vi "SetGetUnits - Test.vi"() -> ()   [LabVIEW 2017]
uses:
  AT901 API/Structures/Struct SystemUnits.ctl
  AT901 API/TypeDefinitions/ES_LengthUnit.ctl
  AT901 API/TypeDefinitions/ES_AngleUnit.ctl
  AT901 API/TypeDefinitions/ES_TemperatureUnit.ctl
  AT901 API/TypeDefinitions/ES_PressureUnit.ctl
  AT901 API/TypeDefinitions/ES_HumidityUnit.ctl
panel:
  in  "SystemUnits 2":T1
  out "SystemUnits":T1
  out "error out":errorcluster
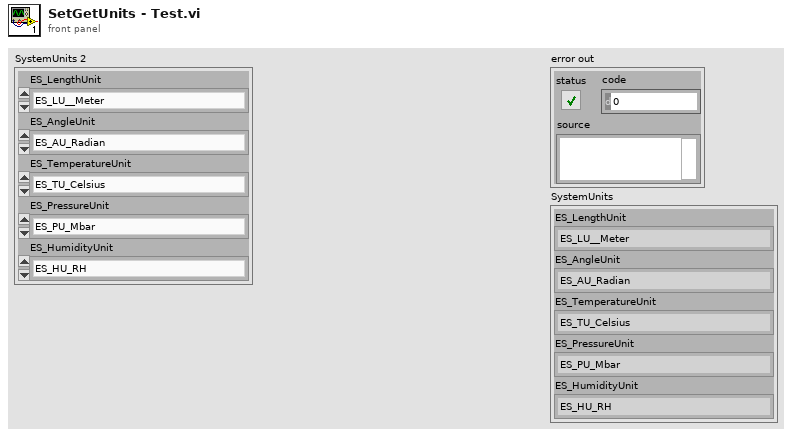
[diagram p1: front panel]
types:
  T1 = typedef "Struct SystemUnits.ctl" = cluster{"ES_LengthUnit":T2, "ES_AngleUnit":T3, "ES_TemperatureUnit":T4, "ES_PressureUnit":T5, "ES_HumidityUnit":T6}
  T2 = typedef "ES_LengthUnit.ctl" = enum32{"ES_LU__Meter", "ES_LU_Millimeter", "ES_LU_Micron", "ES_LU_Foot", "ES_LU_Yard", "ES_LU_Inch"}
  T3 = typedef "ES_AngleUnit.ctl" = enum32{"ES_AU_Radian", "ES_AU_Degree", "ES_AU_Gon"}
  T4 = typedef "ES_TemperatureUnit.ctl" = enum32{"ES_TU_Celsius", "ES_TU_Fahrenheit"}
  T5 = typedef "ES_PressureUnit.ctl" = enum32{"ES_PU_Mbar", "ES_PU_HPascal", "ES_PU_KPascal", "ES_PU_MmHg", "ES_PU_Psi", "ES_PU_InH2O", "ES_PU_InHg"}
  T6 = typedef "ES_HumidityUnit.ctl" = enum32{"ES_HU_RH"}
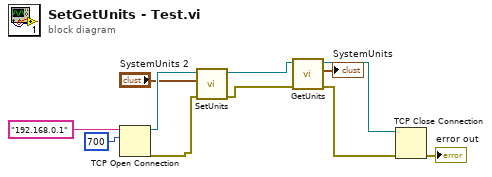
[diagram p0: block diagram]
diagram:
  n1 = TCP Open Connection(address="192.168.0.1", remote port or service name=u16 700) -> (connection ID=w3:refnum<k5>, error out=w8:errorcluster)  [unwired: 3 in]
  n2 = call "SetUnits.vi"("error in (no error)"=w8, "SystemUnits"="SystemUnits 2", "TCP Network Connection in"=w3) -> ("error out"=w7:errorcluster, "TCP Network Connection out"=w4:refnum<k5>)  [unwired: 5 in, 2 out]
  n3 = call "GetUnits.vi"("error in (no error)"=w7, "TCP Network Connection in"=w4) -> ("error out"=w6:errorcluster, "SystemUnits"=→"SystemUnits":T1, "TCP Network Connection out"=w5:refnum<k5>)  [unwired: 5 in, 2 out]
  n4 = TCP Close Connection(connection ID=w5, error in (no error)=w6) -> (error out=→"error out":errorcluster)  [unwired: 1 in, 1 out]
